vi "Write Teller.vi"(10 "Teller":refnum<class "Teller.lvclass">, 11 "Msg in":refnum<class "Msg.lvclass">) -> (3 "Msg out":refnum<class "Msg.lvclass">)   [LabVIEW 2025, in "jettl.lvlib" / "Msg.lvclass"]
uses:
  Msg.lvclass
  Teller/Teller.lvclass
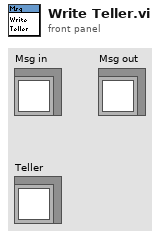
[diagram p1: front panel]
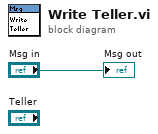
[diagram p0: block diagram]
diagram:
  "Msg out" <- "Msg in"
